vi "Gasliste erweitern.vi"(9 "Aktuelle Gasliste FT-IR":T1[](array[typedef])) -> (1 "Gasliste gesamt":T1[](array[typedef]))   [LabVIEW 2020, in "FT-IR.lvlib"]
uses:
  FT-IR.lvlib
  Visualisierungs Elemente/String - Ausgabefeld.ctl
  Algebraic Modul/FGV Algebraic Aktionen.ctl
  Analysator Definition/FGV Analysator Definition Aktionen.ctl
  AK-Schnittstelle/AK Namen Aktionen.ctl
  Linearisierung V2/Aktionen Polynom Daten speichern.ctl
  Log Konfig/Log Sequence FGV Aktion.ctl
  Algebraic Modul/Algebraic Modul.lvlib
  Analysator Definition/Analysator Definition.lvlib
  AK-Schnittstelle/AK-Schnittstelle.lvlib
  Linearisierung V2/Linearisierung v2.lvlib
  Log Konfig/LogKonfig.lvlib
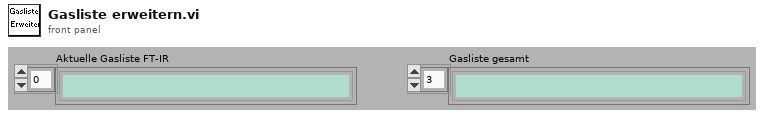
[diagram p1: front panel]
types:
  T1 = typedef "String - Ausgabefeld.ctl" = string
  T2 = typedef "LogKonfig.lvlib/Log Sequence FGV Aktion.ctl" = enum16{"initialisieren", "lesen", "schreiben", "laden", "speichern", "übertragen"}
  T3 = typedef "Linearisierung v2.lvlib/Aktionen Polynom Daten speichern.ctl" = enum16{"lesen", "laden", "speichern", "schreiben", "schreiben alle", "Liste erstellen", "aktivieren", "deaktivieren", "aktiv abfragen"}
  T4 = typedef "AK-Schnittstelle.lvlib/AK Namen Aktionen.ctl" = enum16{"lesen", "laden", "speichern Namen", "AK Namen", "Liste erstellen", "EKFG erstellen", "speichern EKFG", "EKFG schreiben", "Neuen Eintrag erzeugen"}
  T5 = typedef "Analysator Definition.lvlib/FGV Analysator Definition Aktionen.ctl" = enum16{"lesen", "MB setzen", "MB KAL setzen", "laden"}
  T6 = typedef "FT-IR.lvlib/Algebraic Modul.lvlib/FGV Algebraic Aktionen.ctl" = enum16{"lesen", "laden", "speichern", "berechnen", "schreiben"}
  T7 = typedef "Analysator Definition.lvlib/Betriebsdaten Komponente.ctl" = cluster{"Namen":string[], "MB Namen":string[], "Einheit":string, "MB Aktuell":u16, "MB Endwert":u16, "CalGase":u16[], "MB für KAL":u16[], "CG für KAL":u16[]}
  T8 = cluster{"Index Array":i32[], "Namen Array":string[], "Spektrum File Name":bool}
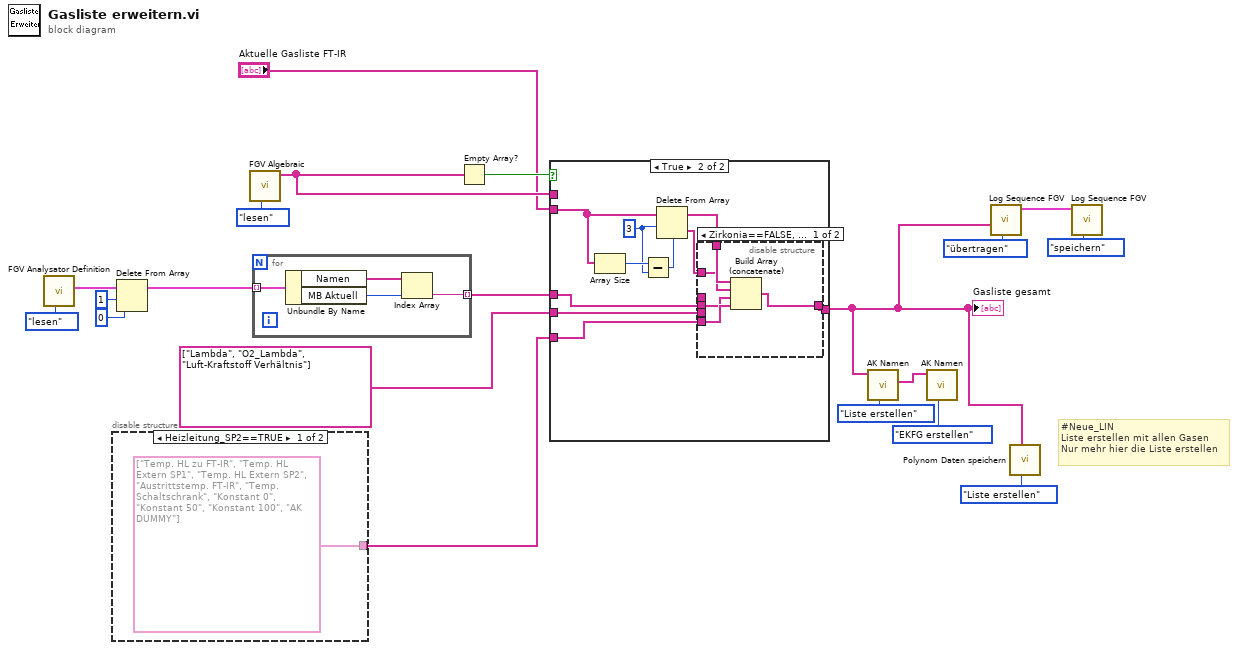
[diagram p0: block diagram]
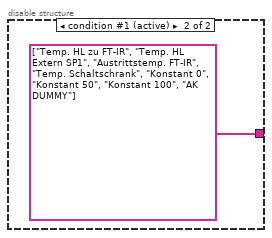
[diagram p2: hidden frame]
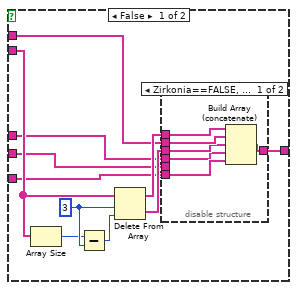
[diagram p3: hidden frame]
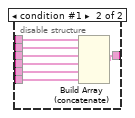
[diagram p4: hidden frame]
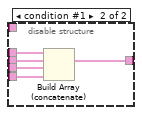
[diagram p5: hidden frame]
diagram:
  # "#Neue_LIN \nListe erstellen mit allen Gasen\nNur mehr hier die Liste erstellen"
  n1 = call "FGV Analysator Definition.vi"("Aktionen"=FGV_Analysator_Definition_Aktionen."lesen") -> ("Betriebsdaten"=w15:T7[])  [unwired: 6 in, 4 out]
  n2 = disable-structure shown="Heizleitung_SP2==TRUE" {
    disable-tunnel: [string[] ["Temp. HL zu FT-IR", "Temp. HL Extern SP1", "Temp. HL Extern SP2", "Austrittstemp. FT-IR", "Temp. Schaltschrank", "Konstant 0", "Konstant 50", "Konstant 100", "AK DUMMY"] ("Namen") string[] ["Temp. HL zu FT-IR", "Temp. HL Extern SP1", "Austrittstemp. FT-IR", "Temp. Schaltschrank", "Konstant 0", "Konstant 50", "Konstant 100", "AK DUMMY"] ("Namen")] -> w17
    frame condition #0 {
    }
    frame condition #1 (active) {
    }
  }
  n3 = Delete From Array(array=w15, length=1 ("Länge"), index=0 ("Index")) -> (array with subset deleted=w5:T7[])  [unwired: 1 out]
  n4 = call "FGV Algebraic.vi"("Aktionen Algebraic"=FGV_Algebraic_Aktionen."lesen") -> ("Namen"=w20:string[])  [unwired: 6 in, 4 out]
  n5 = for {
    tunnel: w5 -> [w26] mode=indexing
    tunnel: [w23] -> w12 mode=indexing
    n6 = Unbundle By Name(w26) -> ("Namen"=w25:string[], "MB Aktuell"=w24:u16)
    n7 = Index Array(array=w25, index=w24) -> (element=w23:string)
  }
  n8 = Empty Array?(array=w20) -> (empty?=w18:bool)
  n9 = case shown="True" w18 {
    tunnel: [w32 w60] -> w1
    tunnel: w17 -> [w29 w59]
    tunnel: "Aktuelle Gasliste FT-IR" -> [w34 w53]
    tunnel: w20 -> [w31 _]
    tunnel: w12 -> [w28 w58]
    tunnel: string[] ["Lambda", "O2_Lambda", "Luft-Kraftstoff Verhältnis"] ("Namen") -> [w27 w57]
    frame False {
      w37 = 3 ("Länge")
      n10 = Array Size(array=w34) -> (size(s)=w35:i32)
      n11 = Subtract(x=w35, y=w37) -> (x-y=w36:i32)
      n12 = Delete From Array(array=w34, length=w37, index=w36) -> (deleted portion=w30:T1[], array with subset deleted=w33:T1[])
      n13 = disable-structure shown="Zirkonia==FALSE, Standard" {
        disable-tunnel: w33 -> [w43 w50]
        disable-tunnel: [w42 w49] -> w32
        disable-tunnel: w31 -> [w41 w48]
        disable-tunnel: w30 -> [w40 w47]
        disable-tunnel: w29 -> [w39 w46]
        disable-tunnel: w28 -> [w38 w45]
        disable-tunnel: w27 -> [_ w44]
        frame condition #0 (active) {
          n14 = Build Array (concatenate)(w43, w41, w40, w38, w39) -> (w42:T1[])
        }
        frame condition #1 {
          n15 = Build Array (concatenate)(w50, w48, w47, w45, w44, w46) -> (w49:T1[])
        }
      }
    }
    frame True {
      w54 = 3 ("Länge")
      n16 = Array Size(array=w53) -> (size(s)=w55:i32)
      n17 = Subtract(x=w55, y=w54) -> (x-y=w56:i32)
      n18 = Delete From Array(array=w53, length=w54, index=w56) -> (deleted portion=w51:T1[], array with subset deleted=w52:T1[])
      n19 = disable-structure shown="Zirkonia==FALSE, Standard" {
        disable-tunnel: [w65 w70] -> w60
        disable-tunnel: _ -> [_ w69]
        disable-tunnel: w59 -> [w64 w67]
        disable-tunnel: w58 -> [w63 w68]
        disable-tunnel: w57 -> [_ w66]
        disable-tunnel: w52 -> [w62 _]
        disable-tunnel: w51 -> [w61 _]
        frame condition #0 (active) {
          n20 = Build Array (concatenate)(w62, w61, w63, w64) -> (w65:T1[])
        }
        frame condition #1 {
          n21 = Build Array (concatenate)(w69, w68, w66, w67) -> (w70:string[])
        }
      }
    }
  }
  "Gasliste gesamt" <- w1
  n22 = call "AK Namen.vi"("Aktionen"=AK_Namen_Aktionen."Liste erstellen", "Aktuelle Gasliste FT-IR"=w1) -> ("Namen"=w8:string[])  [unwired: 6 in, 3 out]
  n23 = call "AK Namen.vi"("Aktionen"=AK_Namen_Aktionen."EKFG erstellen", "Aktuelle Gasliste FT-IR"=w8) -> ()  [unwired: 6 in, 4 out]
  n24 = call "Log Sequence FGV.vi"("Aktion"=Log_Sequence_FGV_Aktion."übertragen", "Neue Gasliste gesamt"=w1) -> ("Cluster (out)"=w2:T8)  [unwired: 9 in]
  n25 = call "Polynom Daten speichern.vi"("Aktionen"=Aktionen_Polynom_Daten_speichern."Liste erstellen", "Aktuelle Gasliste FT-IR"=w1) -> ()  [unwired: 4 in, 6 out]
  n26 = call "Log Sequence FGV.vi"("Aktion"=Log_Sequence_FGV_Aktion."speichern", "Cluster (in)"=w2) -> ()  [unwired: 9 in, 1 out]
